vi "Battery Waveforms.vi"(10 "Log Read Data":cluster{refnum<class "RDS State.lvclass">[]}[](array[cluster]), 11 "Header":T1) -> (2 "Log Data Out":cluster{refnum<class "RDS State.lvclass">[]}[](array[cluster]), 3 "Header Out":T1, 5 "Battery WFs":waveform(dbl)[](array[waveform]))   [LabVIEW 2015, in "Log Waveform Processors.lvlib"]
uses:
  Log Waveform Processors.lvlib
  RDS State Tracker/RDS State/RDS State.lvclass
  Actors/RDS Logger Actor/RDS Logger Actor/RDS Logger Actor/Logger Header.ctl
  RDS State Tracker/RDS State/RDS State.lvclass/RDS State.ctl
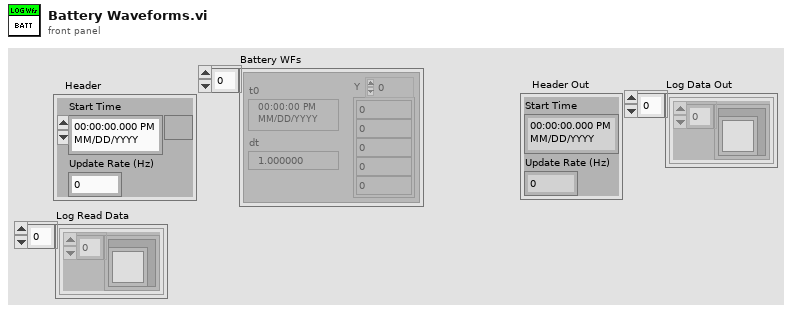
[diagram p1: front panel]
types:
  T1 = typedef "Log Waveform Processors.lvlib/Logger Header.ctl" = cluster{"Start Time":timestamp, "Update Rate (Hz)":dbl}
  T2 = typedef "RDS Instrument Library.lvlib/Battery Data.ctl" = cluster{"Battery Status":T3, "Pack Voltage":sgl, "Pack Current":sgl, "Pack Capacity":sgl, "Max Cell Temp":sgl, "Min Cell Temp":sgl, "Max Cell Voltage":sgl, "Min Cell Voltage":sgl}
  T3 = typedef "RDS Instrument Library.lvlib/Battery Status.ctl" = enum16{"Pack Normal", "Alarm: Cell temp too high", "Alarm: Pack voltage too high", "Warn: Pack voltage too high ", "Alarm: Pack voltage too low", "Warn: Pack voltage low", "Alarm Pack current too high", "Warn: Pack current too high ", "Fault: Pack to chassis connection detected", "Fault: Pack to cell connection error", "Fautl: System error"}
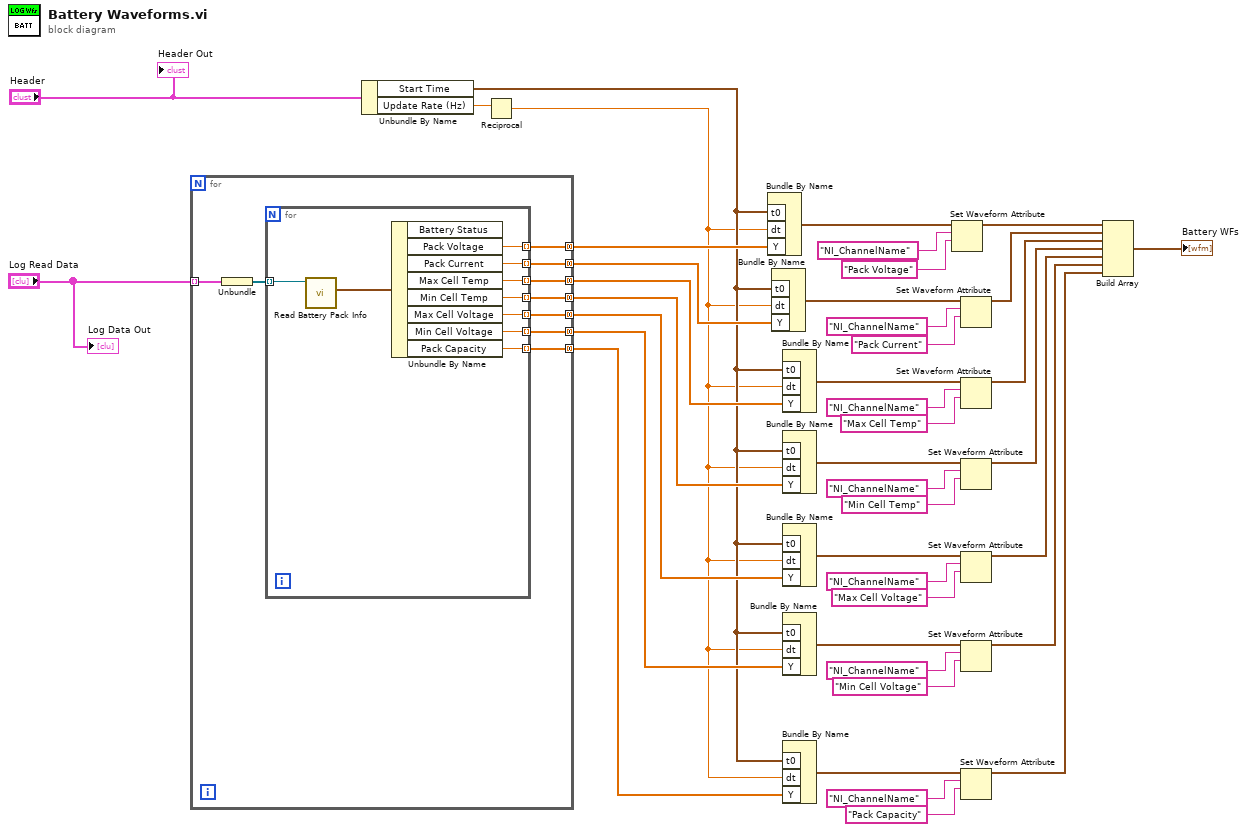
[diagram p0: block diagram]
diagram:
  n1 = for {
    tunnel: "Log Read Data" -> [w50] mode=indexing
    tunnel: [w48] -> w12 mode=concatenating
    tunnel: [w47] -> w17 mode=concatenating
    tunnel: [w46] -> w18 mode=concatenating
    tunnel: [w45] -> w34 mode=concatenating
    tunnel: [w44] -> w35 mode=concatenating
    tunnel: [w43] -> w38 mode=concatenating
    tunnel: [w42] -> w3 mode=concatenating
    n2 = Unbundle(w50) -> (w49:refnum<class "RDS State.lvclass">[])
    n3 = for {
      tunnel: w49 -> [w52] mode=indexing
      tunnel: [w58] -> w48 mode=indexing
      tunnel: [w57] -> w47 mode=indexing
      tunnel: [w56] -> w46 mode=indexing
      tunnel: [w55] -> w45 mode=indexing
      tunnel: [w54] -> w44 mode=indexing
      tunnel: [w53] -> w43 mode=indexing
      tunnel: [w51] -> w42 mode=indexing
      n4 = call "Read Battery Pack Info.vi"("RDS State in"=w52) -> ("Battery Pack Info"=w59:T2)  [unwired: 8 in, 2 out]
      n5 = Unbundle By Name(w59) -> ("Pack Voltage"=w58:sgl, "Pack Current"=w57:sgl, "Max Cell Temp"=w56:sgl, "Min Cell Temp"=w55:sgl, "Max Cell Voltage"=w54:sgl, "Min Cell Voltage"=w53:sgl, "Pack Capacity"=w51:sgl)  [unwired: 1 out]
    }
  }
  n6 = Unbundle By Name("Header") -> ("Start Time"=w5:timestamp, "Update Rate (Hz)"=w9:dbl)
  n7 = Reciprocal(x=w9) -> (1/x=w4:dbl)
  n8 = Bundle By Name("t0"=w5, "dt"=w4, "Y"=w12) -> (w13:waveform(sgl))  [unwired: 1 in]
  n9 = Bundle By Name("t0"=w5, "dt"=w4, "Y"=w17) -> (w15:waveform(sgl))  [unwired: 1 in]
  n10 = Bundle By Name("t0"=w5, "dt"=w4, "Y"=w18) -> (w16:waveform(sgl))  [unwired: 1 in]
  n11 = Bundle By Name("t0"=w5, "dt"=w4, "Y"=w34) -> (w30:waveform(sgl))  [unwired: 1 in]
  n12 = Bundle By Name("t0"=w5, "dt"=w4, "Y"=w35) -> (w31:waveform(sgl))  [unwired: 1 in]
  n13 = Bundle By Name("t0"=w5, "dt"=w4, "Y"=w38) -> (w37:waveform(sgl))  [unwired: 1 in]
  n14 = Bundle By Name("t0"=w5, "dt"=w4, "Y"=w3) -> (w6:waveform(sgl))  [unwired: 1 in]
  n15 = Set Waveform Attribute(5:"Pack Voltage" ("name"), 6:"NI_ChannelName" ("name"), 7:w13) -> (3:w19:waveform(sgl))  [unwired: 1 in, 2 out]
  n16 = Set Waveform Attribute(5:"Pack Current" ("name"), 6:"NI_ChannelName" ("name"), 7:w15) -> (3:w20:waveform(sgl))  [unwired: 1 in, 2 out]
  n17 = Set Waveform Attribute(5:"Max Cell Temp" ("name"), 6:"NI_ChannelName" ("name"), 7:w16) -> (3:w21:waveform(sgl))  [unwired: 1 in, 2 out]
  n18 = Set Waveform Attribute(5:"Min Cell Temp" ("name"), 6:"NI_ChannelName" ("name"), 7:w30) -> (3:w39:waveform(sgl))  [unwired: 1 in, 2 out]
  n19 = Set Waveform Attribute(5:"Max Cell Voltage" ("name"), 6:"NI_ChannelName" ("name"), 7:w31) -> (3:w40:waveform(sgl))  [unwired: 1 in, 2 out]
  n20 = Set Waveform Attribute(5:"Min Cell Voltage" ("name"), 6:"NI_ChannelName" ("name"), 7:w37) -> (3:w41:waveform(sgl))  [unwired: 1 in, 2 out]
  n21 = Set Waveform Attribute(5:"Pack Capacity" ("name"), 6:"NI_ChannelName" ("name"), 7:w6) -> (3:w1:waveform(sgl))  [unwired: 1 in, 2 out]
  n22 = Build Array(w19, w20, w21, w39, w40, w41, w1) -> (→"Battery WFs":waveform(sgl)[])
  "Header Out" <- "Header"
  "Log Data Out" <- "Log Read Data"
